vi "flow rate(pump control).vi"(4 "State":i16, 5 "Time":dbl format="%.2f", 6 "Sensor Values":dbl[](array[numeric]), 7 "Set Points":dbl[](array[numeric])) -> (0 "required data":T1={"Set Point names"=["pump control", "Tubing size code"], "required number of setpoints"=2, "required number of sensors"=0, "Sensor names"=[]}, 3 "output value":dbl)   [LabVIEW 2019]
panel:
  in  "pumpflow":dbl[unit][](array[numeric])=[9.549296547316535e-09, 3.342253804929783e-08, 1.2732395447351617e-07, 2.705634032562094e-07, 4.4563384065730255e-07, 6.04788783748884e-07] format="%.3f"
  in  "tubing size":enum16{"13", "14", "16", "25", "17", "18"}(ring)
  # "Enter the correct information for this control code in the required data structure below. Then make the current value default by right clicking on the border of the data structure."
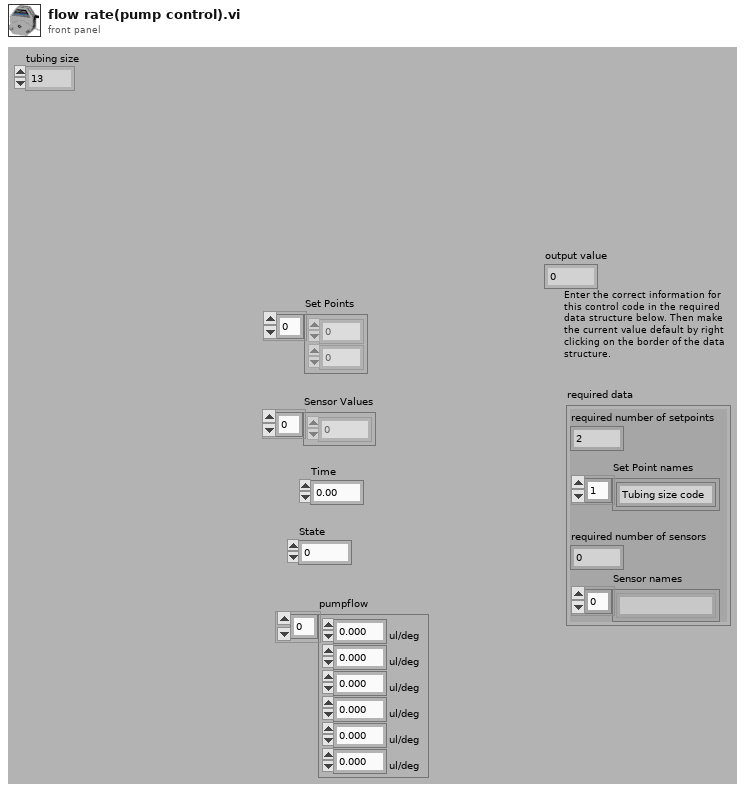
[diagram p1: front panel]
types:
  T1 = cluster{"Set Point names":string[], "required number of setpoints":u8, "required number of sensors":u8, "Sensor names":string[]}
  T2 = cluster{"Set Points[0]":dbl, "Set Points[1]":dbl}
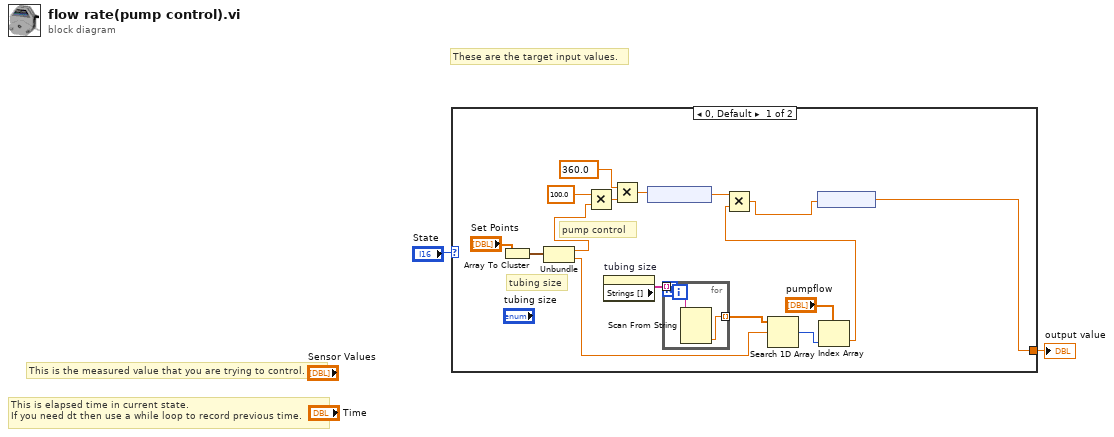
[diagram p0: block diagram]
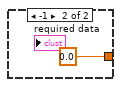
[diagram p2: hidden frame]
diagram:
  # "These are the target input values."
  # "This is the measured value that you are trying to control."
  # "This is elapsed time in current state.\nIf you need dt then use a while loop to record previous time."
  n1 = case shown="0, Default" "State" {
    tunnel: [w3 0.0 ("fraction on")] -> w1
    frame 0, Default {
      # "tubing size"
      # "pump control"
      n2 = Array To Cluster(array="Set Points") -> (cluster=w18:T2)
      n3 = Unbundle(w18) -> ("Set Points[0]"=w11:dbl, "Set Points[1]"=w12:dbl)
      n4 = Multiply(x=100.0, y=w11) -> (x*y=w9:dbl)
      n5 = property on="tubing size" class="Enum (strict)"() -> ("Strings []"=w15:string[])  [unwired: 2 in, 2 out]
      n6 = Multiply(x=360.0 ("y"), y=w9) -> (x*y=w7:dbl)
      n7 = node(w7) -> (w6:dbl[unit])
      n8 = for {
        tunnel: w15 -> [w20] mode=indexing
        tunnel: [w19] -> w17 mode=indexing
        n9 = Scan From String(input string=w20) -> (output 1=w19:dbl)  [unwired: 4 in, 3 out]
      }
      n10 = Search 1D Array(1D array=w17, element=w12) -> (index of element=w13:i32)  [unwired: 1 in]
      n11 = Index Array(array="pumpflow", index=w13) -> (element=w5:dbl[unit])
      n12 = Multiply(x=w6, y=w5) -> (x*y=w4:dbl[unit])
      n13 = node(w4) -> (w3:dbl)
    }
    frame -1 {
    }
  }
  "output value" <- w1
